vi "Write Groups.vi"(8 "error in (no error)":errorcluster, 10 "Groups":refnum<data-value>, 11 "Blackboard in":refnum<class "Blackboard.lvclass">) -> (0 "error out":errorcluster, 3 "Blackboard out":refnum<class "Blackboard.lvclass">)   [LabVIEW 2021, in "Blackboard.lvclass"]
uses:
  Blackboard.lvclass
  Support/Data DVR Type.ctl
  Support/Tags Map Type.ctl
  Support/Status Type.ctl
  Support/Data Type.ctl
  Support/Group Map Type.ctl
  Blackboard.lvclass/Blackboard.ctl
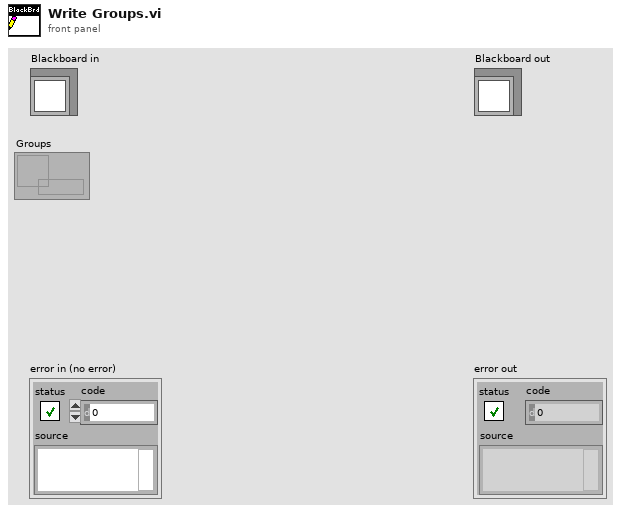
[diagram p1: front panel]
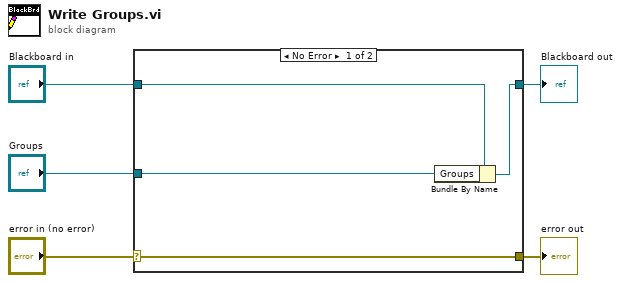
[diagram p0: block diagram]
diagram:
  n1 = case shown="No Error" "error in (no error)" {
    selector: "error in (no error)" -> [w9 w10]
    tunnel: [w9 w10] -> w4
    tunnel: [w7 w11] -> w2
    tunnel: "Blackboard in" -> [w8 w11]
    tunnel: "Groups" -> [w6 _]
    frame No Error {
      n2 = Bundle By Name(cluster=w8, "Groups"=w6) -> (w7:refnum<class "Blackboard.lvclass">)
    }
    frame Error {
    }
  }
  "error out" <- w4
  "Blackboard out" <- w2
